vi "Directory to Text file Compare FTP.vi"(6 "error in (no error)":errorcluster, 8 "delimiter (\\t)":string=",", 9 "File datastore Path IN":path, 10 "File Pattern (*.CSV .ddf)":string, 11 "Directory Path":path) -> (0 "Number of files Unmanaged":i32, 2 "Unmanaged Files":string[](array[string]), 4 "error out":errorcluster)   [LabVIEW 2011]
uses:
  <vilib>/Utility/file.llb/Read From Spreadsheet File (string).vi
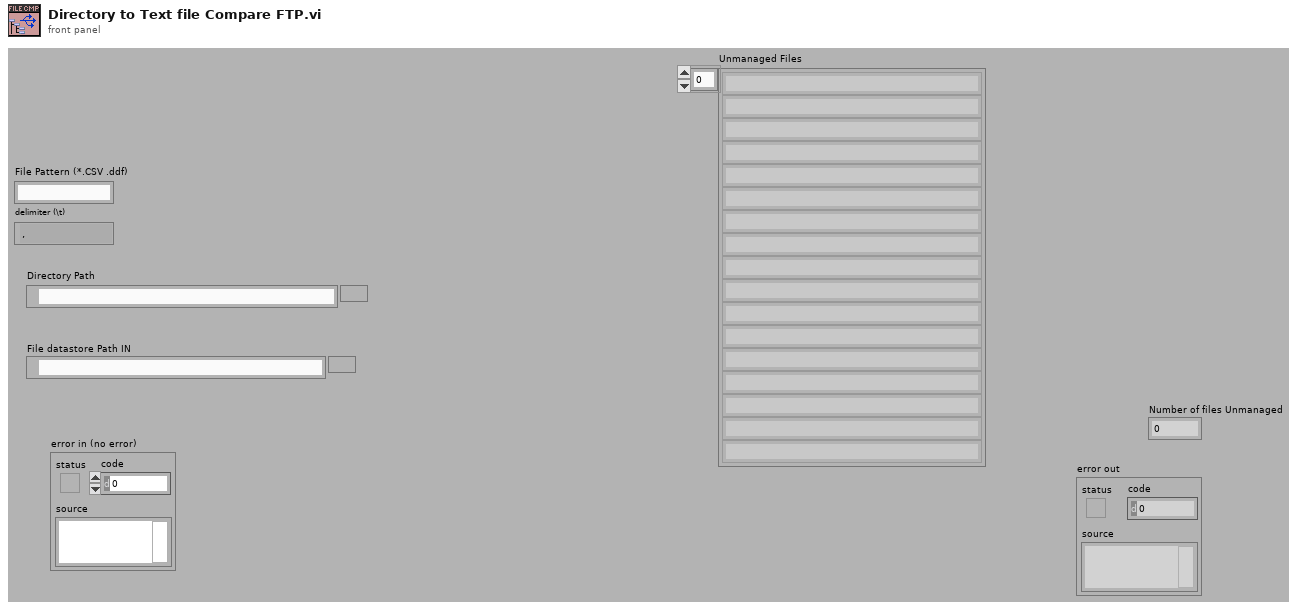
[diagram p1: front panel]
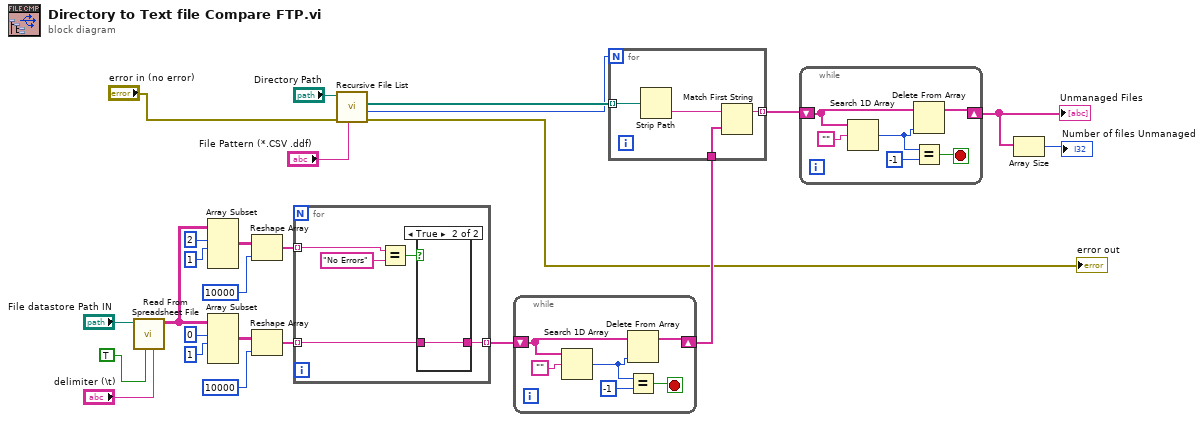
[diagram p0: block diagram]
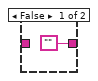
[diagram p2: hidden frame]
diagram:
  n1 = call-poly <vilib>:"Read From Spreadsheet File.vi"("delimiter (\\t)"="delimiter (\\t)", "transpose (no:F)"=TRUE, "file path (dialog if empty)"="File datastore Path IN") -> ("all rows"=w14:string[][])  [unwired: 4 in, 4 out]
  n2 = Array Subset(array=w14, index (row)=2 ("index"), length (row)=1 ("length")) -> (w9:string[][])  [unwired: 2 in]
  n3 = Array Subset(array=w14, index (row)=0 ("index"), length (row)=1 ("length")) -> (w8:string[][])  [unwired: 2 in]
  n4 = Reshape Array(w9, 10000 ("dimension size")) -> (w12:string[])
  n5 = Reshape Array(w8, 10000 ("dimension size")) -> (w13:string[])
  n6 = for {
    tunnel: w12 -> [w30] mode=indexing
    tunnel: w13 -> [w27] mode=indexing
    tunnel: [w26] -> w7 mode=indexing
    n7 = Equal?(x=w30, y="No Errors") -> (x = y?=w28:bool)
    n8 = case shown="True" w28 {
      tunnel: w27 -> [_ w32]
      tunnel: ["" w32] -> w26
      frame False {
      }
      frame True {
      }
    }
  }
  n9 = call <vilib>:"Recursive File List.vi"("pattern"="File Pattern (*.CSV .ddf)", "error in (no error)"="error in (no error)", "Folder Path"="Directory Path") -> ("error out"=→"error out":errorcluster, "Number of Files"=w19:i32, "All Files in Dir"=w23:path[])  [unwired: 4 in, 2 out]
  n10 = while {
    shift-right: [w33] -> w6
    shift-left: w7 -> [w35]
    stop <- w36 stop-if-true
    n11 = Search 1D Array(1D array=w35, element="") -> (index of element=w34:i32)  [unwired: 1 in]
    n12 = Delete From Array(array=w35, index=w34) -> (array with subset deleted=w33:string[])  [unwired: 1 in, 1 out]
    n13 = Equal?(x=w34, y=-1) -> (x = y?=w36:bool)
  }
  n14 = for {
    N: w19 -> [_]
    tunnel: w23 -> [w42] mode=indexing
    tunnel: [w40] -> w5 mode=indexing
    tunnel: w6 -> [w39]
    n15 = Strip Path(path=w42) -> (name=w41:string)  [unwired: 1 out]
    n16 = Match First String(2:w39, 3:w41) -> (1:w40:string)  [unwired: 1 out]
  }
  n17 = while {
    shift-right: [w43] -> w4
    shift-left: w5 -> [w45]
    stop <- w46 stop-if-true
    n18 = Search 1D Array(1D array=w45, element="") -> (index of element=w44:i32)  [unwired: 1 in]
    n19 = Delete From Array(array=w45, index=w44) -> (array with subset deleted=w43:string[])  [unwired: 1 in, 1 out]
    n20 = Equal?(x=w44, y=-1) -> (x = y?=w46:bool)
  }
  "Unmanaged Files" <- w4
  n21 = Array Size(array=w4) -> (size(s)=→"Number of files Unmanaged":i32)
